vi "UpdateRPMData.vi"(5 "Pulse Params":T1={"Amplitude"=5.0, "Duty Cycle"=0.1, "Shape"=enum."Square"}, 6 "error in (no error)":errorcluster, 7 "Noise StdDev":dbl=0.05 format="%.2p", 8 "RPM":dbl=0.1, 9 "Refnum in":refnum<k21>) -> (0 "error out":errorcluster, 1 "Waveform":waveform(dbl)(graph), 2 "RPM out":dbl=0.1, 3 "Refnum out":refnum<k21>)   [LabVIEW 2014]
uses:
  <vilib>/DAQmx/write.llb/DAQmx Write (Analog Wfm 1Chan NSamp).vi
  <resource>/objmgr/daqmx.rc
  <vilib>/measure/NI_MABase.lvlib
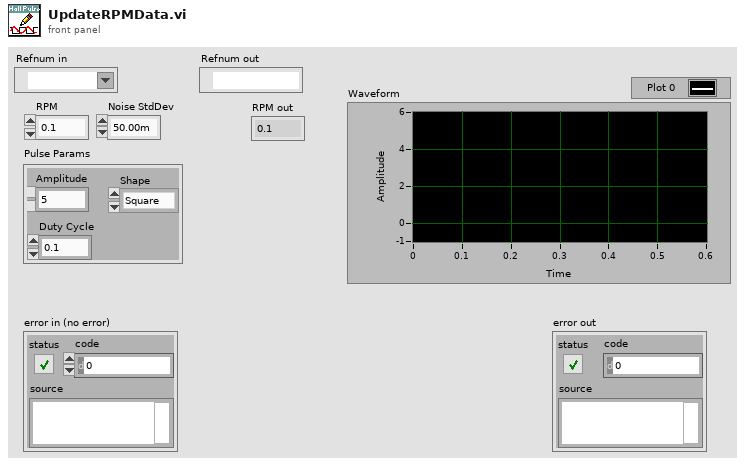
[diagram p1: front panel]
types:
  T1 = cluster{"Amplitude":dbl, "Duty Cycle":dbl, "Shape":enum16{"Square", "Cosine"}}
  T2 = cluster{"SampClk.Rate":dbl, "SampQuant.SampPerChan":dbl}
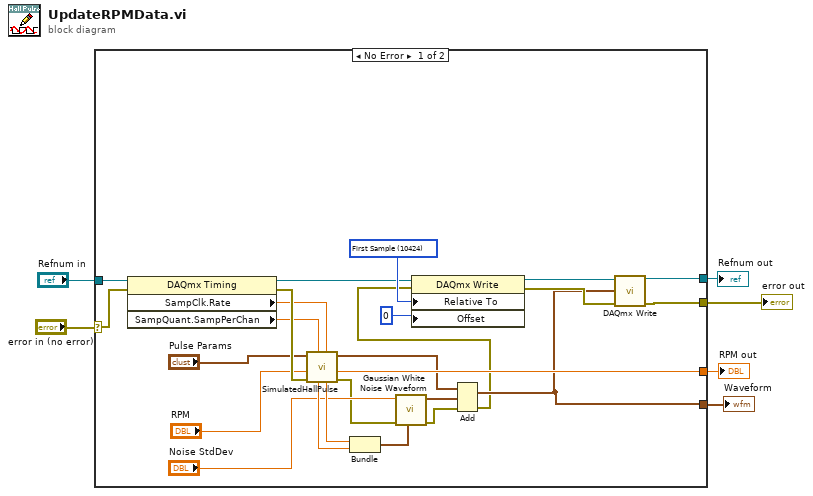
[diagram p0: block diagram]
diagram:
  n1 = case shown="No Error" "error in (no error)" {
    selector: "error in (no error)" -> [w22 w31]
    tunnel: [w26 w31] -> w6
    tunnel: [w25 w30] -> w5
    tunnel: "Refnum in" -> [w23 w30]
    tunnel: [w18 _] -> w2
    tunnel: [w11 _] -> w1
    frame No Error {
      w24 = 10424 items=["First Sample"=10424, "Current Write Position"=10430] ("RelativeTo")
      n2 = property class="DAQmx Timing"(reference=w23, error in=w22) -> (reference out=w19:refnum<k21>, error out=w21:errorcluster, "SampClk.Rate"=w17:dbl, "SampQuant.SampPerChan"=w16:dbl)
      n3 = call "SimulatedHallPulse.vi"("AO Rate"=w17, "Buffer Size"=w16, "error in (no error)"=w21, "RPM"="RPM", "Pulse Params"="Pulse Params") -> ("error out"=w10:errorcluster, "RPM out"=w18:dbl, "Waveform Graph"=w12:waveform(dbl))  [unwired: 2 in]
      n4 = Bundle("SampClk.Rate"=w17, "SampQuant.SampPerChan"=w16) -> (w15:T2)  [unwired: 1 in]
      n5 = call <vilib>:"Gaussian White Noise Waveform.vi"("sampling info"=w15, "error in (no error)"=w10, "standard deviation"="Noise StdDev") -> ("error out"=w9:errorcluster, "signal out"=w13:waveform(dbl))  [unwired: 7 in]
      n6 = Add(1:w13, 2:w12, 4:w9) -> (0:w11:waveform(dbl), 3:w8:errorcluster)
      n7 = property class="DAQmx Write"(reference=w19, error in=w8, "Relative To"=w24, "Offset"=0) -> (reference out=w27:refnum<k21>, error out=w28:errorcluster)
      n8 = call-poly <vilib>:"DAQmx Write.vi"("task/channels in"=w27, "data"=w11, "error in"=w28) -> ("task out"=w25:refnum<k21>, "error out"=w26:errorcluster)  [unwired: 10 in, 1 out]
    }
    frame Error {
    }
  }
  "error out" <- w6
  "Refnum out" <- w5
  "RPM out" <- w2
  "Waveform" <- w1
